vi "optionsAcq_spectralRange_waveNr.vi"(0 "reference":refnum<class "OSA.lvclass">, 1 "range min (waveNr)":sgl, 2 "range max (waveNr)":sgl, 3 "write action":enum16{"range min", "range max", "both"}(ring), 4 "readWrite":enum16{"read", "write"}(ring), 5 "error in (no error)":errorcluster) -> (14 "duplicate reference":refnum<class "OSA.lvclass">, 15 "range min read (waveNr)":sgl, 16 "range max read (waveNr)":sgl, 19 "error out":errorcluster)   [LabVIEW 2010, in "OSA.lvclass"]
doc: "optionsAcq_spectralRange_waveNr enables a reduction of the spectrum dataset size while maintaining resolution. This is done by calling the functions 'FTS_SetAcquisitionOption_MinWaveNr' and 'FTS_SetAcquisitionOption_MaxWaveNr' with the desired wavenumber range. \n\nNotice that this cutting is done during the calculation of the spectrum from the interferogram and does not affect the interferogram at all, nor the time required to perform a measurement, (spectra update time unchanged).\n\nA smaller spectrum dataset can also be obtained by switching to low resolution mode. \n\nIn write mode; the spectrum graph x range will be updated accordingly, (plot_spectrum.vi will update graph with new range). This applies to spectrum graph which reference has been wired to init.vi., (see tree.vi for compatible graph).\n\nIn write both mode; the range min and max will be swapped if min being larger than max."
uses:
  OSA.lvclass
  OSA20X_misc.lvlib
  FTSLib.dll
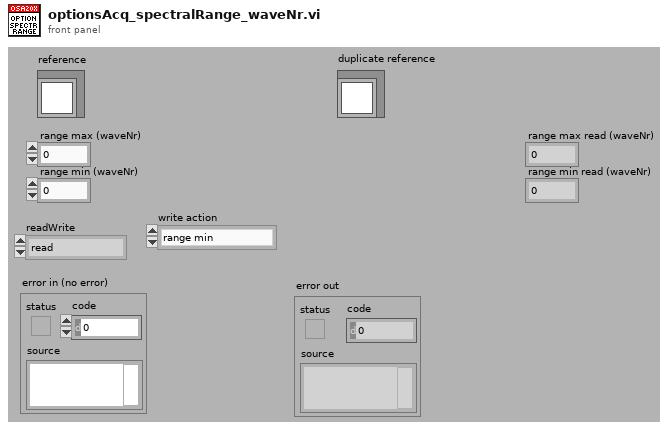
[diagram p1: front panel]
types:
  T1 = typedef "OSA.lvclass/ObjectAttributes.ctl" = cluster{"Stop":bool, "dataType":T2, "spectrometerIdx":u16, "buffer size interferogram":i32, "interferogram":cluster{"new":bool, "plot_x_ min":sgl, "plot_x_max":sgl, "plot_y_min":sgl, "plot_y_max":sgl, "Graph Intrfrgrm":T3, "timeStamp":u32, "signal (%)":dbl, "traces":cluster{"idx":u32, "broadBand":bool, "monoChromatic":bool, "peakToPeakSignal":dbl, "peakToPeakPos":dbl}[], "traces idx last":i32}, "spectrum":cluster{"new":bool, "plot_x_min":sgl, "plot_x_max":sgl, "plot_unit_x":T4, "plot_unit_y":T5, "plot_y_min":sgl, "plot_y_max":sgl, "Graph Spectrum":T3, "timeStamp":u32, "X_VAL_OPTIONS":enum16{"MIN_MAX", "ARRAY"}, "traces":cluster{"idx":u32}[], "traces idx last":i32}, "Thorlabs_OSA_64.lvclass:queue_action.ctlqueue ref":refnum<queue>, "action":T6, "plot zoom step":dbl, "buffer semaphore":T7, "acq stopped":bool, "dataType active":T2, "temperature (degr C)":sgl, "pressure (hPa)":sgl, "rel humidity (%)":sgl, "settings":cluster{"resolution":T8, "sensitivity":T9, "Average":bool, "average nr":u32, "apodisation":T10, "acq delay (ms)":u32, "airMesure":T11, "wmtr on":bool, "intfgrm_smooth_width":u16, "intfgrm_smooth_nrOfPasses":u16, "intfgrm_smooth":T12, "phaseCorrection":T13, "zeroFill":u8, "spectr_smooth":T12, "spectr_smooth_width":u16, "spectr_smooth_nrOfPasses":u16, "resolution (/cm)":sgl, "REF wavelength, (nm)":dbl, "gain_idx":u16, "gainAuto":bool, "gain_relative":dbl, "PD sensitivity mode":T14, "PD senseMode implemented":bool, "SensorTemperature implemented":bool, "SensorPressure implemented":bool, "SensorHumidity implemented":bool}, "peaks position":sgl[], "peaks width":sgl[], "peaks height":sgl[], "peaks max nr":u32, "peaks latest nr":i32, "peaks new":bool, "power":dbl, "power new":bool, "path":string, "wavelength (WNr)":dbl, "wavelength new":bool, "buffer size spectrum":i32, "status":string, "VI reference":refnum<vi>, "funcPointer":u64, "libraryPointer":u64, "singleAcquisition":bool, "coherenceLength (cm)":dbl, "coherenceLength new":bool, "spectrometer model":string, "spectrometer serial nr":string, "peaks thld left":sgl[], "peaks thld right":sgl[], "coherenceLength error (cm)":dbl, "ADC bits":u16, "peaks position centroid":sgl[], "peaks height centroid":sgl[], "OSA series":T15, "channel index (all)":u16}
  T2 = typedef "OSA.lvclass/acq_dataType.ctl" = enum16{"none", "interferogram", "spectrum"}
  T3 = typedef "OSA.lvclass/graph_intensity.ctl" = refnum<vi>
  T4 = typedef "OSA.lvclass/spectrum_x_unit.ctl" = enum16{"wavenr/cm", "THz", "eV", "nm_air", "nm_vac"}
  T5 = typedef "OSA.lvclass/y_unit.ctl" = enum16{"ADC counts", "dBm pwr absolute", "dBm pwr density", "mW pwr absolute", "mW pwr density"}
  T6 = typedef "OSA.lvclass/queue_action.ctl" = enum16{"none", "stop", "GUI_plotInterferogram", "GUI_plotSpectrum", "GUI_plotInterferogramRescale", "GUI_plotSpectrumRescale", "GUI_plotInterferogramReset", "GUI_plotSpectrumReset", "GUI_plotInterferogramAutoScaleY", "GUI_plotSpectrumAutoScaleY", "GUI_plotInterferogramZoomOut", "GUI_plotSpectrumZoomOut", "GUI_plotInterferogramPane", "GUI_plotSpectrumPane", "GUI_plotInterferogramZoomMouse", "GUI_plotSpectrumZoomMouse", "ENVIRONMENT temperature", "ENVIRONMENT pressure", "MODE_resolution set", "MODE_resolution get", "MODE_sensitivity set", "MODE_sensitivity get", "MODE_PDTemperature set", "MODE_PDTemperature get", "REBOOT/RESET firmware", "ACQASYNC_acquireSingleSpectrum", "ACQASYNC_continuous start", "ACQASYNC_continuous stop\n", "ACQASYNC_get last interferogram", "ACQASYNC_get last spectrum", "ACQASYNC_get last waveNr", "ACQOPT_interferogram smoothing set", "ACQOPT_interferogram smoothing get", "ACQOPT_spectrum smoothing set", "ACQOPT_spectrum smoothing get", "ACQOPT_apodisation type set", "ACQOPT_apodisation type get", "ACQOPT_phase correction type set", "ACQOPT_phase correction type get", "ACQOPT_acqIntervall_set", "ACQOPT_acqIntervall_get", "ACQOPT_average spectrum set", "ACQOPT_average spectrum get", "ACQOPT_rolling average set", "ACQOPT_rolling average get", "ACQOPT_zero fill factor set", "ACQOPT_zero fill factor get", "ACQOPT_cycle counting set", "ACQOPT_cycle counting get", "ACQOPT_air measure option set", "ACQOPT_air measure option get", "ACQOPT_gainLevel auto get", "ACQOPT_gainLevel auto set", "ACQOPT_gainLevel get", "ACQOPT_gainLevel set", "ACQOPT_getAll", "INSTRUMENT_PROPERTY_range_WaveNr_min", "INSTRUMENT_PROPERTY_range_WaveNr_max", "INSTRUMENT_PROPERTY_reference_wavelength_cm^-1", "INSTRUMENT_PROPERTY_samplesPerRefPeriod", "INSTRUMENT_PROPERTY_resolution_waveNrPercm", "INSTRUMENT_PROPERTY_availableGainLevels", "INSTRUMENT_PROPERTY_status", "CONVERT", "ANALYSE_POWER", "ANALYSE_PEAKS", "ANALYSE_WAVELENGTH", "ANALYSE_SPECTRUM", "ANALYSE_INTERFEROGRAM", "ANALYSE_COHERENCE_LENGTH", "MATH", "MATH_power", "MATH_peaks", "FILE", "miscellaneous"}
  T7 = typedef "Semaphore RefNum" = refnum<k1>
  T8 = typedef "OSA.lvclass/resolution.ctl" = enum16{"low", "high"}
  T9 = typedef "OSA.lvclass/sensitivityMode.ctl" = enum16{"low", "low medium", "high medium", "high"}
  T10 = typedef "OSA.lvclass/apodisation.ctl" = enum16{"NONE", "NORTON_BEER_WEAK", "NORTON_BEER_MEDIUM", "NORTON_BEER_STRONG", "TRIANGULAR", "COSINE", "HANN", "HAMMING", "BLACKMANHARRIS3", "BLACKMANHARRIS4", "GAUSSIAN"}
  T11 = typedef "OSA.lvclass/airMeasure.ctl" = enum16{"TEMPERATURE", "PRESSURE"}
  T12 = typedef "OSA.lvclass/smoothing.ctl" = enum16{"NONE", "BINOMIAL", "SAVITSKY_GOLAY", "FOURIER", "MOVING_AVERAGE", "GAUSSIAN"}
  T13 = typedef "OSA.lvclass/phaseCorrection.ctl" = enum16{"NONE", "MERTZ", "FORMAN", "MERTZ_FILE", "FORMAN_FILE", "FUTURE COMP."}
  T14 = typedef "OSA.lvclass/PDTemperatureMode.ctl" = enum16{"cool: better sensitivity/noise floor", "warm: extended wl range"}
  T15 = typedef "OSA_series.ctl" = enum16{"OSA200", "OSA300", "UNKNOWN"}
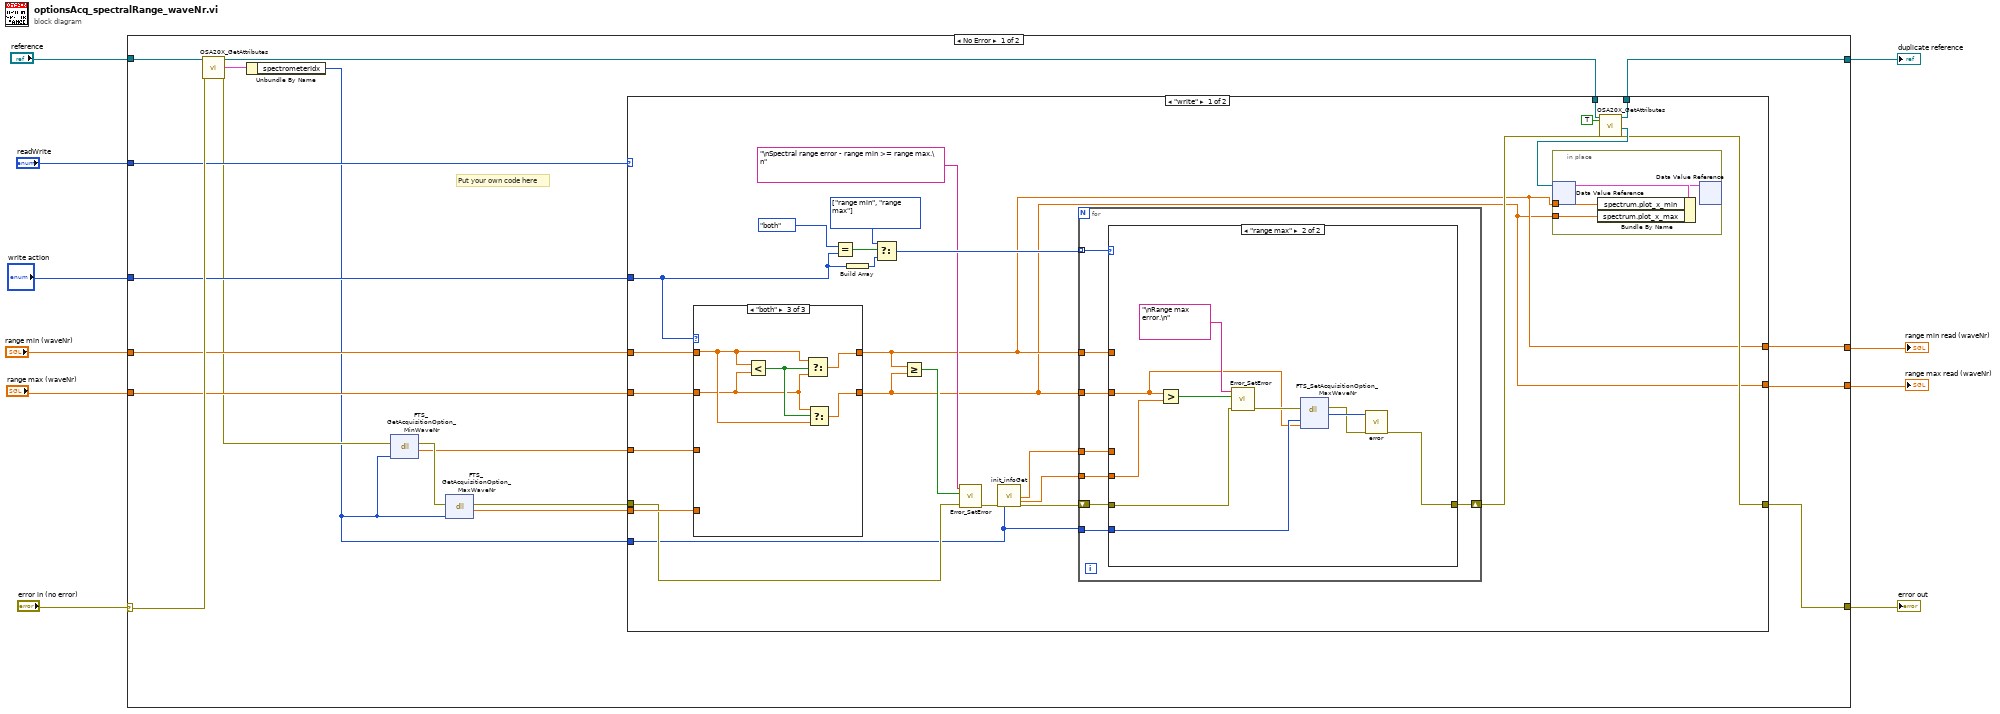
[diagram p0: block diagram]
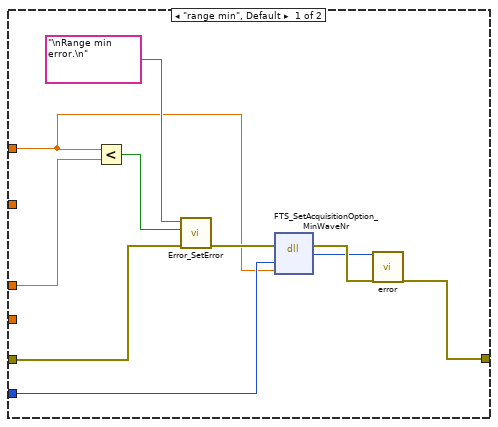
[diagram p4: hidden frame]
diagram:
  n1 = case shown="No Error" "error in (no error)" {
    selector: "error in (no error)" -> [w27 w102]
    tunnel: [w11 w102] -> w10
    tunnel: "reference" -> [w28 w103]
    tunnel: [w15 w103] -> w7
    tunnel: "range max (waveNr)" -> [w25 w100]
    tunnel: "write action" -> [w23 _]
    tunnel: "range min (waveNr)" -> [w24 w101]
    tunnel: "readWrite" -> [w22 _]
    tunnel: [w13 w101] -> w2
    tunnel: [w12 w100] -> w1
    frame No Error {
      # "Put your own code here"
      n2 = call "OSA20X_GetAttributes.vi"("reference in"=w28, "error in (no error)"=w27) -> ("reference out"=w16:refnum<class "OSA.lvclass">, "Data"=w26:T1, "error out"=w20:errorcluster)  [unwired: 14 in, 1 out]
      n3 = Unbundle By Name(w26) -> ("spectrometerIdx"=w14:u16)
      n4 = dll-call lib="FTSLib.dll" fn="FTS_GetAcquisitionOption_MinWaveNr"(error in=w20, "spectrIdx"=w14) -> (error out=w21:errorcluster, "return type"=w18:sgl)  [unwired: 3 in, 1 out]
      n5 = dll-call lib="FTSLib.dll" fn="FTS_GetAcquisitionOption_MaxWaveNr"(error in=w21, "spectrIdx"=w14) -> (error out=w19:errorcluster, "return type"=w17:sgl)  [unwired: 3 in, 1 out]
      n6 = case shown="\"write\"" w22 {
        tunnel: w25 -> [w45 _]
        tunnel: w24 -> [w43 _]
        tunnel: w19 -> [w41 w99]
        tunnel: w23 -> [w46 _]
        tunnel: [w34 w99] -> w11
        tunnel: w18 -> [w44 w97]
        tunnel: w17 -> [w42 w96]
        tunnel: w16 -> [w33 w98]
        tunnel: [w32 w98] -> w15
        tunnel: w14 -> [w31 _]
        tunnel: [w30 w97] -> w13
        tunnel: [w29 w96] -> w12
        frame "write" {
          w50 = enum16{"range min", "range max", "both"}[] [enum."range min", enum."range max"] items=["range min", "range max", "both"]
          n7 = case shown="\"both\"" w46 {
            tunnel: w45 -> [_ w62 w65]
            tunnel: [w59 w62 w63] -> w29
            tunnel: [w60 w61 w64] -> w30
            tunnel: w44 -> [_ w61 _]
            tunnel: w43 -> [w60 _ w66]
            tunnel: w42 -> [w59 _ _]
            frame "range min", Default {
            }
            frame "range max" {
            }
            frame "both" {
              n8 = Less?(x=w66, y=w65) -> (x < y?=w67:bool)
              n9 = Select(t=w66, s=w67, f=w65) -> (s? t:f=w64:sgl)
              n10 = Select(t=w65, s=w67, f=w66) -> (s? t:f=w63:sgl)
            }
          }
          n11 = Equal?(x=enum16{"range min", "range max", "both"}."both" ("action"), y=w46) -> (x = y?=w51:bool)
          n12 = Build Array(w46) -> (w49:enum16{"range min", "range max", "both"}[])
          n13 = Select(t=w50, s=w51, f=w49) -> (s? t:f=w48:enum16{"range min", "range max", "both"}[])
          n14 = Greater Or Equal?(x=w30, y=w29) -> (x >= y?=w39:bool)
          n15 = call "Error_SetError.vi"("error in"=w41, "status (true)"=w39, "source(\"\")"="\nSpectral range error - range min >= range max.\n" ("source(\"\")")) -> ("error out"=w40:errorcluster)  [unwired: 4 in]
          n16 = call "init_infoGet.vi"("error in (no error)"=w40, "spectrIdx"=w31) -> ("waveNrMin"=w54:sgl, "waveNrMax"=w53:sgl, "error out"=w47:errorcluster)  [unwired: 14 in, 1 out]
          n17 = for {
            tunnel: w54 -> [w75]
            tunnel: w53 -> [w74]
            tunnel: w30 -> [w73]
            tunnel: w29 -> [w72]
            tunnel: w48 -> [w71] mode=indexing
            tunnel: w31 -> [w70]
            shift-right: [w68] -> w35
            shift-left: w47 -> [w69]
            n18 = case shown="\"range max\"" w71 {
              tunnel: w69 -> [w84 w92]
              tunnel: w75 -> [w85 _]
              tunnel: w74 -> [_ w93]
              tunnel: w73 -> [w79 _]
              tunnel: w72 -> [_ w86]
              tunnel: w70 -> [w81 w90]
              tunnel: [w77 w87] -> w68
              frame "range min", Default {
                n19 = Less?(x=w79, y=w85) -> (x < y?=w83:bool)
                n20 = call "Error_SetError.vi"("error in"=w84, "status (true)"=w83, "source(\"\")"="\nRange min error.\n" ("source(\"\")")) -> ("error out"=w80:errorcluster)  [unwired: 4 in]
                n21 = dll-call lib="FTSLib.dll" fn="FTS_SetAcquisitionOption_MinWaveNr"(error in=w80, "spectrIdx"=w81, "waveNr_min"=w79) -> (error out=w78:errorcluster, "return type"=w76:i32)  [unwired: 4 in, 1 out]
                n22 = call "error.vi"("result code"=w76, "error in (no error)"=w78) -> ("error out"=w77:errorcluster)  [unwired: 15 in, 2 out]
              }
              frame "range max" {
                n23 = Greater?(x=w86, y=w93) -> (0:w91:bool)
                n24 = call "Error_SetError.vi"("error in"=w92, "status (true)"=w91, "source(\"\")"="\nRange max error.\n" ("source(\"\")")) -> ("error out"=w94:errorcluster)  [unwired: 4 in]
                n25 = dll-call lib="FTSLib.dll" fn="FTS_SetAcquisitionOption_MaxWaveNr"(error in=w94, "spectrIdx"=w90, "waveNr_min"=w86) -> (error out=w88:errorcluster, "return type"=w89:i32)  [unwired: 4 in, 1 out]
                n26 = call "error.vi"("result code"=w89, "error in (no error)"=w88) -> ("error out"=w87:errorcluster)  [unwired: 15 in, 2 out]
              }
            }
          }
          n27 = call "OSA20X_GetAttributes.vi"("reference in"=w33, "OnlyGetDvrReference(False)"=TRUE, "error in (no error)"=w35) -> ("reference out"=w32:refnum<class "OSA.lvclass">, "DataRef"=w37:refnum<data-value>, "error out"=w34:errorcluster)  [unwired: 13 in, 1 out]
          n28 = in-place {
            in-place-border: w30 -> [w56]
            in-place-border: w29 -> [w55]
            n29 = in-place-dvr #1(w37) -> (w58:T1)  [unwired: 1 out]
            n30 = Bundle By Name(cluster=w58, "spectrum.plot_x_min"=w56, "spectrum.plot_x_max"=w55) -> (w57:T1)
            n31 = in-place-dvr #1(w57) -> ()  [unwired: 2 out]
          }
        }
        frame "read" {
        }
      }
    }
    frame Error {
      # "Error"
    }
  }
  "error out" <- w10
  "duplicate reference" <- w7
  "range max read (waveNr)" <- w1
  "range min read (waveNr)" <- w2
